vi "AutoParameter Guidance Omega.vi"(2 "error in":errorcluster, 3 "eta_last":dbl[](array[numeric])=[0.0, 0.0, 0.0, 0.0, 0.0, 0.0], 4 "eta_ref":dbl[](array[numeric])=[0.0, 0.0, 0.0, 0.0, 0.0, 0.0]) -> (0 "error out":errorcluster, 1 "Omega":T1=[[1.0, 0.0, 0.0, 0.0, 0.0, 0.0], [0.0, 1.0, 0.0, 0.0, 0.0, 0.0], [0.0, 0.0, 1.0, 0.0, 0.0, 0.0], [0.0, 0.0, 0.0, 0.0, 0.0, 0.0], [0.0, 0.0, 0.0, 0.0, 0.0, 0.0], [0.0, 0.0, 0.0, 0.0, 0.0, 1.0]] caption="Real Matrix")   [LabVIEW 2012]
uses:
  <vilib>/Analysis/Matrix/Datatypes/RealMatrix.ctl
  <vilib>/imath/engines/lvmath2/RunTimeEngine/ErrorHandling/NIMS_Finalize Error.vi
  <vilib>/imath/engines/lvmath2/RunTimeEngine/Managers/WorkSpace/UID Generator.vi
  <vilib>/imath/engines/lvmath2/RunTimeEngine/ArithmeticOperatorToken/NIMS_ArithmeticOperator_minus.vi
  <instcachedir>/0/NIMS_ArithmeticOperator_minus_E353D3D62E0E432C853B0E64BA14CDF8.lvgen/NIMS_ArithmeticOperator_minus_E353D3D62E0E432C853B0E64BA14CDF8_003.vi
  <vilib>/imathl/engines/lvmath/Functions/Error Handling/Create Error.vi
  <vilib>/Analysis/Matrix/Numeric/Conversions/Array To Matrix - RA2.vi
  <vilib>/imath/engines/lvmath2/RunTimeEngine/Managers/SymbolTable/Clear UID.vi
  <vilib>/imath/engines/lvmath2/RunTimeEngine/NodeEndStatement/NIMS_NodeEndStatement_Output.vi
  <instcachedir>/0/NIMS_NodeEndStatement_Output_53EC0D466D134D7ABD903AC30B43404B.lvgen/NIMS_NodeEndStatement_Output_53EC0D466D134D7ABD903AC30B43404B_016.vi
  <vilib>/imath/engines/lvmath2/RunTimeEngine/BuiltInFunctions/abs/NIMS_abs(signed).vi
  <instcachedir>/0/NIMS_abs(signed)_C4FCB8E6058B49B797C7C8D53CA5F6EC.lvgen/NIMS_abs(signed)_C4FCB8E6058B49B797C7C8D53CA5F6EC_001.vi
  <vilib>/imath/engines/lvmath2/RunTimeEngine/RangeToken/NIMS_Range_R2 - Integer.vi
  <instcachedir>/0/NIMS_Range_R2 - Integer_CD92A44154CA48D58B2F3E711AB114DB.lvgen/NIMS_Range_R2 - Integer_CD92A44154CA48D58B2F3E711AB114DB_000.vi
  <vilib>/imath/engines/lvmath2/RunTimeEngine/CommandStatement/MC_CommandStatement_break.vi
  <vilib>/imath/engines/lvmath2/RunTimeEngine/VariableToken/Read/NIMS_Get Elements - RV(_) - Check.vi
  <instcachedir>/0/NIMS_Get Elements - RV(_) - Check_09E565EE58C54071A799578B82C9999A.lvgen/NIMS_Get Elements - RV(_) - Check_09E565EE58C54071A799578B82C9999A_000.vi
  <vilib>/imath/engines/lvmath2/RunTimeEngine/ReplaceToken/NIMS_Replace - Check Linear.vi
  <instcachedir>/0/NIMS_Replace - Check Linear_44ABB4D6A819426DBDF25CCE6827BF1D.lvgen/NIMS_Replace - Check Linear_44ABB4D6A819426DBDF25CCE6827BF1D_001.vi
  <vilib>/imath/engines/lvmath2/RunTimeEngine/ReplaceToken/NIMS_Replace - Size Check _(_)=S.vi
  <instcachedir>/0/NIMS_Replace - Size Check _(_)=S_5AC8AA27B9694BB9828B57BCF666F597.lvgen/NIMS_Replace - Size Check _(_)=S_5AC8AA27B9694BB9828B57BCF666F597_000.vi
  <vilib>/imath/engines/lvmath2/RunTimeEngine/ReplaceToken/NIMS_Replace - V(S)=S.vi
  <instcachedir>/0/NIMS_Replace - V(S)=S_927EF1B21AA84780A9A306EC96B904EC.lvgen/NIMS_Replace - V(S)=S_927EF1B21AA84780A9A306EC96B904EC_000.vi
  <vilib>/imath/engines/lvmath2/RunTimeEngine/RunTimeType/NIMS_RunTimeType_From StrictType (excl LVString).vi
  <instcachedir>/0/NIMS_RunTimeType_From StrictType (excl LVString)_AC52D965D0864706932D20A05968E122.lvgen/NIMS_RunTimeType_From StrictType (excl LVString)_AC52D965D0864706932D20A05968E122_000.vi
  <vilib>/imath/engines/lvmath2/RunTimeEngine/LocalVariableDefStatement/MC_LocalVariableDefStatement_Display.vi
  <vilib>/imath/engines/lvmath2/RunTimeEngine/ErrorHandling/NIMS_Create Error From Enums.vi
  <vilib>/imath/engines/lvmath2/RunTimeEngine/VariableToken/Read/NIMS_Get Elements - CV(_) - Check.vi
  <instcachedir>/0/NIMS_Get Elements - CV(_) - Check_9400805D97754C2091B853F6E24C0606.lvgen/NIMS_Get Elements - CV(_) - Check_9400805D97754C2091B853F6E24C0606_001.vi
  <vilib>/imath/engines/lvmath2/RunTimeEngine/BuiltInFunctions/diag/NIMS_diag.vi
  <instcachedir>/0/NIMS_diag_1CFEA6743F82472F8CC957F2917D2329.lvgen/NIMS_diag_1CFEA6743F82472F8CC957F2917D2329_004.vi
  <vilib>/Analysis/Matrix/NI_Matrix.lvlib
  <vilib>/imath/engines/lvmath2/RunTimeEngine/Managers/SymbolTable/NIMS_WorkSpace.lvlib
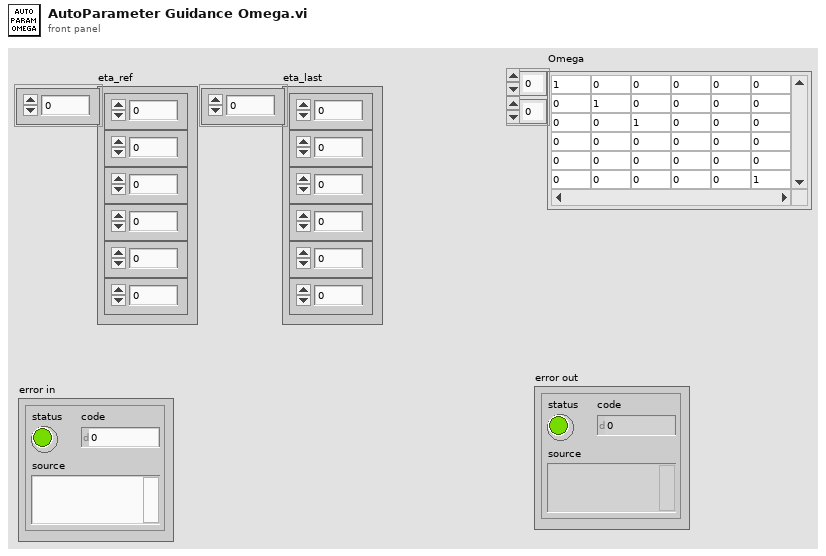
[diagram p1: front panel]
types:
  T1 = typedef "NI_Matrix.lvlib/RealMatrix.ctl" = dbl[][]
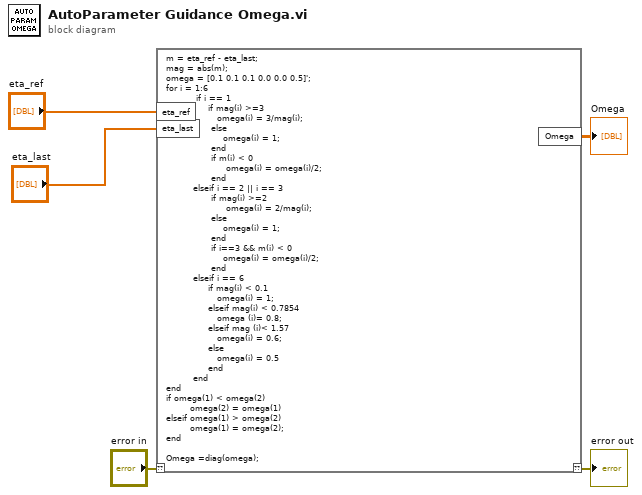
[diagram p0: block diagram]
diagram:
  n1 = mathscript code="m = eta_ref - eta_last;\nmag = abs(m);\nomega = [0.1 0.1 0.1 0.0 0.0 0.5]';\nfor i = 1:6\n          if i == 1\n              if mag(i) >=3\n                 omega(i) = 3/mag(i);\n               else \n                   omega(i) = 1;\n               end\n               if m(i) < 0 \n                    omega(i) = omega(i)/2;\n               end\n         elseif i == 2 || i == 3\n               if mag(i) >=2\n                    omega(i) = 2/mag(i);\n               else\n                   omega(i) = 1;\n               end\n               if i==3 && m(i) < 0 \n                   omega(i) = omega(i)/2;\n               end\n         elseif i == 6\n              if mag(i) < 0.1 \n                 omega(i) = 1;\n              elseif mag(i) < 0.7854\n                 omega (i)= 0.8;\n              elseif mag (i)< 1.57\n                 omega(i) = 0.6;\n              else\n                 omega(i) = 0.5\n              end \n         end\nend          \nif omega(1) < omega(2) \n        omega(2) = omega(1)\nelseif omega(1) > omega(2)\n        omega(1) = omega(2);\nend\n\nOmega =diag(omega);"("??"="error in", "eta_last"="eta_last", "eta_ref"="eta_ref") -> ("??"=→"error out":errorcluster, "Omega"=→"Omega":T1)
